vi "draw.vi"(0 "reference":refnum<class "StateTransitionEdge.lvclass">, 1 "graphics":refnum<class "Graphics.lvclass">, 5 "error in (no error)":errorcluster) -> (14 "reference out":refnum<class "StateTransitionEdge.lvclass">, 19 "error out":errorcluster)   [LabVIEW 2020, in "StateTransitionEdge.lvclass"]
doc: "public void draw(Graphics2D g2)"
uses:
  <resource>/Framework/Providers/Open_GDS/UML/StateTransitionEdge_class/StateTransitionEdge.lvclass
  C:/Program Files (x86)/National Instruments/LabVIEW 2020/resource/Framework/Providers/Open_GDS/UML/ClassRelationshipEdge_class/ClassRelationshipEdge.lvclass
  C:/Program Files (x86)/National Instruments/LabVIEW 2020/resource/Framework/Providers/Open_GDS/UML/SegmentedLineEdge_class/SegmentedLineEdge.lvclass
  <resource>/Framework/Providers/Open_GDS/UML/Graphics_class/Graphics.lvclass
  <resource>/Framework/Providers/Open_GDS/UML/BentStyle_class/BentStyle.lvclass
  <resource>/Framework/Providers/Open_GDS/UML/ArrowHead_class/ArrowHead.lvclass
  <resource>/Framework/Providers/Open_GDS/UML/ClassRelationshipEdge_class/ClassRelationshipEdge.lvclass
  <resource>/Framework/Providers/Open_GDS/UML/SegmentedLineEdge_class/SegmentedLineEdge.lvclass
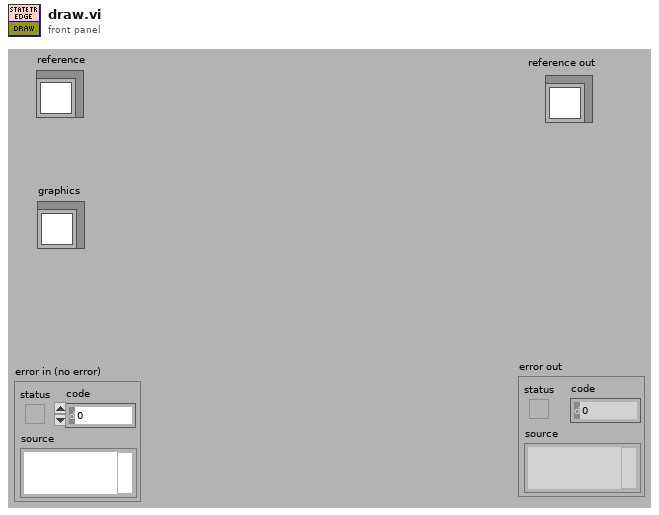
[diagram p1: front panel]
types:
  T1 = typedef "ClassRelationshipEdge.lvclass/ObjectAttributes.ctl" = cluster{"bentStyleRef":refnum<class "BentStyle.lvclass">, "startConnectionOffset":cluster{"x":i32, "y":i32}, "endConnectionOffset":cluster{"x":i32, "y":i32}, "MidLineOffset":cluster{"x":i32, "y":i32}, "DepClass":T2}
  T2 = typedef "ReversedEngineering_ViDependencyDetailsType.ctl" = cluster{"ThisVIs/Ctls":path[], "Dependent_VIs/Ctls":path[]}
  T3 = typedef "SegmentedLineEdge.lvclass/ObjectAttributes.ctl" = cluster{"lineStyle":refnum<class "LineStyle.lvclass">, "startArrowHead":refnum<class "ArrowHead.lvclass">, "endArrowHead":refnum<class "ArrowHead.lvclass">, "startLabel":string, "midLabel":string, "endLabel":string, "MidLabelOffset":T4, "SplitWire":bool}
  T4 = typedef "Point Point2D.ctl" = cluster{"x":dbl, "y":dbl}
  T5 = typedef "BentStyle.lvclass/BentStyleType.ctl" = enum16{"STRAIGHT", "HV", "VH", "HVH", "VHV", "ARC"}
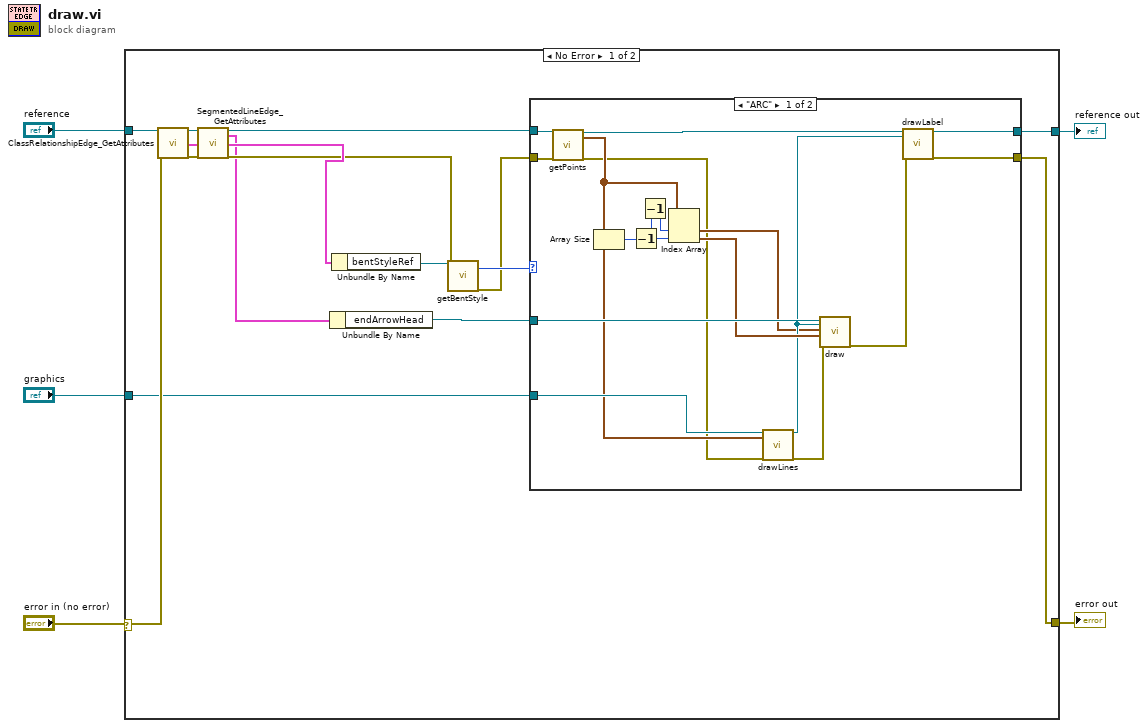
[diagram p0: block diagram]
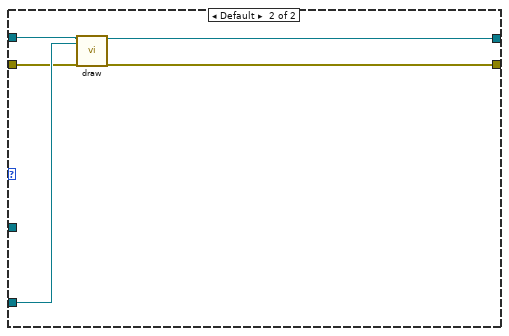
[diagram p2: hidden frame]
diagram:
  n1 = case shown="No Error" "error in (no error)" {
    selector: "error in (no error)" -> [w19 w43]
    tunnel: "reference" -> [w20 w44]
    tunnel: [w16 w43] -> w4
    tunnel: [w15 w44] -> w3
    tunnel: "graphics" -> [w13 _]
    frame No Error {
      n2 = call <resource>:"ClassRelationshipEdge_GetAttributes.vi"("reference in"=w20, "error in (no error)"=w19) -> ("reference out"=w10:refnum<class "StateTransitionEdge.lvclass">, "Data"=w11:T1, "error out"=w9:errorcluster)  [unwired: 14 in, 1 out]
      n3 = call <resource>:"SegmentedLineEdge_GetAttributes.vi"("reference in"=w10, "error in (no error)"=w9) -> ("reference out"=w7:refnum<class "StateTransitionEdge.lvclass">, "Data"=w6:T3, "error out"=w8:errorcluster)  [unwired: 14 in, 1 out]
      n4 = Unbundle By Name(w6) -> ("endArrowHead"=w12:refnum<class "ArrowHead.lvclass">)
      n5 = Unbundle By Name(w11) -> ("bentStyleRef"=w18:refnum<class "BentStyle.lvclass">)
      n6 = call-dynamic "getBentStyle.vi"("reference"=w18, "error in (no error)"=w8) -> ("bentStyle"=w17:T5, "error out"=w14:errorcluster)  [unwired: 15 in, 1 out]
      n7 = case shown="\"ARC\"" w17 {
        tunnel: w7 -> [w36 w42]
        tunnel: w14 -> [w35 w40]
        tunnel: [w27 w39] -> w16
        tunnel: [w29 w38] -> w15
        tunnel: w13 -> [w32 w41]
        tunnel: w12 -> [w37 _]
        frame "ARC" {
          n8 = call-dynamic "getPoints.vi"("reference"=w36, "error in (no error)"=w35) -> ("reference out"=w21:refnum<class "StateTransitionEdge.lvclass">, "points"=w30:T4[], "error out"=w22:errorcluster)  [unwired: 15 in]
          n9 = Array Size(array=w30) -> (size(s)=w34:i32)
          n10 = Decrement(x=w34) -> (x-1=w25:i32)
          n11 = Decrement(x=w25) -> (x-1=w24:i32)
          n12 = Index Array(array=w30, index #1=w24, index #2=w25) -> (element #1=w23:T4, element #2=w33:T4)
          n13 = call <resource>:"drawLines.vi"("reference"=w32, "points"=w30, "error in (no error)"=w22) -> ("reference out"=w26:refnum<class "Graphics.lvclass">, "error out"=w31:errorcluster)  [unwired: 4 in, 11 out]
          n14 = call-dynamic "draw.vi"("reference"=w37, "graphics"=w26, "p1"=w23, "p2"=w33, "error in (no error)"=w31) -> ("error out"=w28:errorcluster)  [unwired: 13 in, 1 out]
          n15 = call <resource>:"drawLabel.vi"("reference"=w21, "graphics"=w26, "error in (no error)"=w28) -> ("reference out"=w29:refnum<class "StateTransitionEdge.lvclass">, "error out"=w27:errorcluster)  [unwired: 15 out]
        }
        frame Default {
          n16 = call-parent "draw.vi"("reference"=w42, "graphics"=w41, "error in (no error)"=w40) -> ("reference out"=w38:refnum<class "StateTransitionEdge.lvclass">, "error out"=w39:errorcluster)  [unwired: 15 in]
        }
      }
    }
    frame Error {
    }
  }
  "reference out" <- w3
  "error out" <- w4
